vi "VI Linearisierung v2.vi"() -> ()   [LabVIEW 2020, in "Linearisierung v2.lvlib"] (continued)
              tunnel: w1175 -> [_ w1180]
              tunnel: w1170 -> [w1177 w1179]
              tunnel: [w1177 w1178] -> w1168
              frame False {
              }
              frame True {
                # "Zeilen von der Tabelle -1"
                n736 = call "Polynom Daten speichern.vi"("Aktionen"=Aktionen_Polynom_Daten_speichern."lesen") -> ("Aktiv"=w1187:bool[])  [unwired: 5 in, 5 out]
                n737 = Array Size(array=w1187) -> (size(s)=w1190:i32)
                n738 = Unbundle(w1179) -> ("Row"=w1193:u32, "Column"=w1192:u32)
                n739 = Subtract(x=w1190, y=29) -> (x-y=w1191:i32)
                n740 = Less Or Equal?(x=w1193, y=w1191) -> (x <= y?=w1194:bool)
                n741 = case shown="True" w1194 {
                  tunnel: w1193 -> [_ w1199]
                  tunnel: [w1197 w1199] -> w1181
                  tunnel: w1191 -> [w1197 _]
                  tunnel: w1192 -> [w1196 w1200]
                  tunnel: [w1195 w1198] -> w1178
                  frame False {
                    n742 = Bundle(w1197, "Column"=w1196) -> (w1195:cluster{i32, "Column":u32})  [unwired: 1 in]
                  }
                  frame True {
                    n743 = Bundle("Row"=w1199, "Column"=w1200) -> (w1198:cluster{"Row":u32, "Column":u32})  [unwired: 1 in]
                  }
                }
                n744 = property on="PolynomTabelleAnzeige" class="Tbl (strikt)"(error in=w1180, "Index Values"=w1178) -> (error out=w1183:errorcluster)  [unwired: 1 in, 1 out]
                n745 = property on="PolynomTabelleEingabe" class="Tbl (strikt)"(error in=w1180, "Index Values"=w1178) -> (error out=w1184:errorcluster)  [unwired: 1 in, 1 out]
                n746 = Build Array(w1181) -> (w1182:u32[])
                n747 = property on="PolynomAktiv" class="Arr"(error in=w1180, "Index Values"=w1182) -> (error out=w1185:errorcluster)  [unwired: 1 in, 1 out]
                n748 = Merge Errors(w1184, w1185, w1183) -> (w1186:errorcluster)
                n749 = call <vilib>:"Clear Errors.vi"("error in (no error)"=w1186) -> ()  [unwired: 5 in, 2 out]
              }
            }
          }
          frame "Spanfaktor" {
            # "#BugFix71"
            n750 = call "Spantabellenanzeige.vi"() -> ("SpanTabelle"=w1204:T48[][])  [unwired: 10 in, 1 out]
            n751 = property on="SpanTabelleEingabe" class="Tbl (strikt)"() -> (error out=w1207:errorcluster, "Index Values"=w1208:T176)  [unwired: 2 in, 1 out]
            n752 = Delete From Array(array=w1204, length=3 ("Länge"), index (col)=0 ("Deaktivierter Index (Spalte)")) -> (deleted portion=w1203:T48[][], array with subset deleted=w1202:T48[][])  [unwired: 1 in]
            n753 = local write "SpanTabelleAnzeige"(w1203) -> ()
            n754 = Not Equal?(x=w1212, y=w1208) -> (x != y?=w1211:cluster{"Row":bool, "Column":bool})
            n755 = Cluster To Array(cluster=w1211) -> (array=w1210:bool[])
            n756 = Or Array Elements(Boolean array=w1210) -> (logical OR=w1209:bool)
            n757 = case shown="True" w1209 {
              tunnel: w1208 -> [w1215 w1220]
              tunnel: w1207 -> [_ w1227]
              tunnel: w1202 -> [_ w1225]
              tunnel: [w1215 w1216] -> w1201
              frame False {
              }
              frame True {
                n758 = Array Size(array=w1225) -> (size(s)=w1219:i32[])
                n759 = Index Array(array=w1219) -> (element=w1218:i32)  [unwired: 1 in]
                n760 = local write "SpanTabelleEingabe"(w1225) -> ()
                n761 = Unbundle(w1220) -> ("Row"=w1223:u32, "Column"=w1222:u32)
                n762 = Subtract(x=w1218, y=29) -> (x-y=w1221:i32)
                n763 = Less Or Equal?(x=w1223, y=w1221) -> (x <= y?=w1224:bool)
                n764 = case shown="True" w1224 {
                  tunnel: w1223 -> [_ w1232]
                  tunnel: [w1230 w1232] -> _
                  tunnel: w1221 -> [w1230 _]
                  tunnel: w1222 -> [w1229 w1233]
                  tunnel: [w1228 w1231] -> w1216
                  frame False {
                    n765 = Bundle(w1230, "Column"=w1229) -> (w1228:cluster{i32, "Column":u32})  [unwired: 1 in]
                  }
                  frame True {
                    n766 = Bundle("Row"=w1232, "Column"=w1233) -> (w1231:cluster{"Row":u32, "Column":u32})  [unwired: 1 in]
                  }
                }
                n767 = property on="SpanTabelleEingabe" class="Tbl (strikt)"("Index Values"=w1216) -> ()  [unwired: 2 in, 2 out]
                n768 = property on="SpanTabelleAnzeige" class="Tbl (strikt)"(error in=w1227, "Index Values"=w1216) -> (error out=w1226:errorcluster)  [unwired: 1 in, 1 out]
                n769 = call <vilib>:"Clear Errors.vi"("error in (no error)"=w1226) -> ()  [unwired: 5 in, 2 out]
              }
            }
          }
        }
        n770 = call "FGV Gasteiler.vi"("Aktionen"=Aktionen_FGV_Gasteiler_Daten."lesen") -> ("Gasteiler Type"=w778:T15, "Anforderung"=w772:bool)  [unwired: 11 in, 6 out]
        n771 = local read "Gasteiler Type"() -> (w764:T15)
        n772 = call "FGV SpanEinstellungen.vi"("Aktion"=Aktion_FGV_SpanEinstellungen."lesen") -> ("automatisch out"=w783:T20)  [unwired: 6 in, 4 out]
        n773 = call "FGV Spans abarbeiten.vi"("Aktion"=Aktion_FGV_Spans_abarbeiten."lesen") -> ("running out"=w766:bool)  [unwired: 5 in, 5 out]
        n774 = call "LIN weiter schalten und Fehlerbehandlung.vi"("Anforderung in"=w772, "automatisch in"=w783, "TestRun"=w782, "Error in"=w770, "Gasteiler Type"=w778, "Referenzen Cluster"=w771, "get Test Data"=w769, "running in"=w766, "Beendet"=w781) -> ("Anforderung out"=w780:bool, "Gasteiler Type out"=w763:T15)  [unwired: 4 in, 1 out]
        n775 = Not Equal?(x=w763, y=w764) -> (x != y?=w765:bool)
        n776 = call "Test Status.vi"("LinV2 läuft"=w766, "Aktion"=Aktion_Test_Status."LinV2") -> ()  [unwired: 10 in, 4 out]
        n777 = case shown="True" w765 {
          tunnel: w763 -> [_ w815]
          frame False {
          }
          frame True {
            # "#HovaCAL_Interference_BugFixes"
            n778 = property on="Gasteiler Type" class="Ring (strikt)"("Val(Sgnl)"=w815) -> (error out=w816:errorcluster)  [unwired: 2 in, 1 out]
            n779 = call <vilib>:"Clear Errors.vi"("error in (no error)"=w816) -> ()  [unwired: 5 in, 2 out]
          }
        }
        n780 = case shown="True" w780 {
          tunnel: w763 -> [_ w823]
          frame False {
            n781 = local write "Störung Kommunikation"(FALSE) -> ()
            n782 = local write "Gasteilerstatus"("" ("Gasteilerstatus")) -> ()
          }
          frame True {
            # "GD Anforderung"
            n783 = case shown="4" w823 {
              frame 0, Default {
                # "LCD Touch Display"
                n784 = call "AK Komm.vi"("Aktionen"=Aktionen_AK_Komm."lesen") -> ("Error"=w826:T17, "Status"=→"Gasteilerstatus":string, "Störung Kommunikation"=w825:bool)  [unwired: 4 in, 4 out]
                "Störung Kommunikation" <- w825
                n785 = Unbundle By Name(w826) -> ("Pressure carrier gas"=w830:bool, "Pressure diluted gas"=w829:bool, "Outlet Pressure"=w828:bool, "SNOX before SAIR"=w827:bool)
                n786 = local write "Error"(w826) -> ()
                n787 = call "FGV Stoerungen sammeln und auswerten.vi"("Aktion"=Aktion_FGV_Stoerungen_sammeln_und_auswerten."lesen") -> ("Errors"=w831:T156)  [unwired: 12 in, 6 out]
                n788 = Bundle By Name(cluster=w831, "Störung Kommunikation"=w825, "Pressure carrier gas"=w830, "Pressure diluted gas"=w829, "Outlet Pressure"=w828, "SNOX before SAIR"=w827) -> (w824:T156)
                n789 = call "FGV Stoerungen sammeln und auswerten.vi"("Errors"=w824, "Aktion"=Aktion_FGV_Stoerungen_sammeln_und_auswerten."error") -> ()  [unwired: 11 in, 7 out]
              }
              frame 1 {
                # "Analog-Display"
                n790 = call "AK Komm_ALT.vi"("Aktionen_ALT"=Aktionen_AK_Komm_ALT."lesen") -> ("Error"=w841:T17, "Status"=w846:string, "Störung Kommunikation"=w842:bool)  [unwired: 6 in, 2 out]
                n791 = Unbundle By Name(w841) -> ("Pressure carrier gas"=w840:bool, "Pressure diluted gas"=w839:bool, "Outlet Pressure"=w838:bool, "SNOX before SAIR"=w837:bool)
                n792 = local write "Gasteilerstatus"(w846) -> ()
                n793 = local write "Störung Kommunikation"(w842) -> ()
                n794 = local write "Error"(w841) -> ()
                n795 = call "FGV Stoerungen sammeln und auswerten.vi"("Aktion"=Aktion_FGV_Stoerungen_sammeln_und_auswerten."lesen") -> ("Errors"=w843:T156)  [unwired: 12 in, 6 out]
                n796 = Bundle By Name(cluster=w843, "Störung Kommunikation"=w842, "Pressure carrier gas"=w840, "Pressure diluted gas"=w839, "Outlet Pressure"=w838, "SNOX before SAIR"=w837) -> (w836:T156)
                n797 = call "FGV Stoerungen sammeln und auswerten.vi"("Errors"=w836, "Aktion"=Aktion_FGV_Stoerungen_sammeln_und_auswerten."error") -> ()  [unwired: 11 in, 7 out]
              }
              frame 2 {
                # "AVL GDU"
                n798 = call "AK Komm.vi"("Aktionen"=Aktionen_AK_Komm."lesen") -> ("Error"=w850:T17, "Status"=w858:string, "Störung Kommunikation"=w849:bool)  [unwired: 4 in, 4 out]
                "Error" <- w850
                n799 = Unbundle By Name(w850) -> ("Pressure carrier gas"=w854:bool, "Pressure diluted gas"=w853:bool, "Outlet Pressure"=w852:bool, "SNOX before SAIR"=w851:bool)
                n800 = local write "Störung Kommunikation"(w849) -> ()
                n801 = local write "Gasteilerstatus"(w858) -> ()
                n802 = call "FGV Stoerungen sammeln und auswerten.vi"("Aktion"=Aktion_FGV_Stoerungen_sammeln_und_auswerten."lesen") -> ("Errors"=w855:T156)  [unwired: 12 in, 6 out]
                n803 = Bundle By Name(cluster=w855, "Störung Kommunikation"=w849, "Pressure carrier gas"=w854, "Pressure diluted gas"=w853, "Outlet Pressure"=w852, "SNOX before SAIR"=w851) -> (w848:T156)
                n804 = call "FGV Stoerungen sammeln und auswerten.vi"("Errors"=w848, "Aktion"=Aktion_FGV_Stoerungen_sammeln_und_auswerten."error") -> ()  [unwired: 11 in, 7 out]
              }
              frame 3 {
                # "Horiba GDC"
                n805 = call "GDC Kom.vi"("Befehl"=Aktion_Befehl."Alarm") -> ("Status (alarm)"=w861:bool, "Fehler"=w863:bool, "Status"=w864:string)  [unwired: 4 in, 4 out]
                "Störung Gasteiler" <- w861
                n806 = local write "Gasteilerstatus"(w864) -> ()
                n807 = local write "Störung Kommunikation"(w863) -> ()
                n808 = call "FGV Stoerungen sammeln und auswerten.vi"("Aktion"=Aktion_FGV_Stoerungen_sammeln_und_auswerten."lesen") -> ("Errors"=w862:T156)  [unwired: 12 in, 6 out]
                n809 = Bundle By Name(cluster=w862, "Störung Kommunikation"=w863, "Störung Gasteiler"=w861) -> (w860:T156)
                n810 = call "FGV Stoerungen sammeln und auswerten.vi"("Errors"=w860, "Aktion"=Aktion_FGV_Stoerungen_sammeln_und_auswerten."error") -> ()  [unwired: 11 in, 7 out]
              }
              frame 4 {
                # "#HovaCALErrors"
                n811 = call "FGV_HovaCAL_Interface_Kommandos.vi"("Aktion"=Aktion_FGV_HovaCAL_Interface_Kommandos."lesen") -> ("connected out ?"=w871:bool)  [unwired: 4 in, 5 out]
                n812 = Not(x=w871) -> (.not. x?=w872:bool)
                n813 = call "FGV Stoerungen sammeln und auswerten.vi"("Aktion"=Aktion_FGV_Stoerungen_sammeln_und_auswerten."lesen") -> ("Errors for AutoSPAN"=w868:T156)  [unwired: 12 in, 6 out]
                n814 = Unbundle By Name(w868) -> ("Störung Kommunikation"=w878:bool, "Pressure carrier gas"=w877:bool, "Pressure diluted gas"=w876:bool, "Outlet Pressure"=w875:bool)
                n815 = case shown="True" w872 {
                  selector: w872 -> [_ w881]
                  tunnel: w868 -> [_ w880]
                  frame False {
                  }
                  frame True {
                    n816 = Bundle By Name(cluster=w880, "Störung Kommunikation"=w881) -> (w882:T156)
                    n817 = call "FGV Stoerungen sammeln und auswerten.vi"("Errors"=w882, "Aktion"=Aktion_FGV_Stoerungen_sammeln_und_auswerten."error") -> ()  [unwired: 11 in, 7 out]
                  }
                }
                n818 = Or(x=w872, y=w878) -> (x .or. y?=w869:bool)
                "Störung Kommunikation 2" <- w869
                n819 = Bundle("Pressure carrier gas"=w877, "Pressure diluted gas"=w876, "Outlet Pressure"=w875, FALSE) -> (w870:T177)  [unwired: 1 in]
                "Error 2" <- w870
                n820 = local write "Störung Kommunikation"(w869) -> ()
                n821 = local write "Error"(w870) -> ()
              }
              frame 5 {
                # "manuell"
              }
            }
          }
        }
        n822 = call "Wertaenderung Systemeinstellungen.vi"("Aktion"=Aktion_Wertaenderung_Gasliste."lesen") -> ("Tests"=w794:T178)  [unwired: 13 in, 1 out]
        n823 = Unbundle By Name(w794) -> ("LinV2 läuft"=w793:bool)
        n824 = case shown="True" w793 {
          selector: w793 -> [_ w820]
          frame False {
          }
          frame True {
            n825 = property on="Systemeinstellung" class="Bool. (strikt)"("Val(Sgnl)"=w820) -> (error out=w819:errorcluster)  [unwired: 2 in, 1 out]
            n826 = call <vilib>:"Clear Errors.vi"("error in (no error)"=w819) -> ()  [unwired: 5 in, 2 out]
          }
        }
        n827 = call "Wertaenderung Gasliste.vi"("Aktion"=Aktion_Wertaenderung_Gasliste."lesen") -> ("Tests"=w791:T178)  [unwired: 13 in, 1 out]
        n828 = Unbundle By Name(w791) -> ("LinV2 läuft"=w790:bool)
        n829 = case shown="True" w790 {
          selector: w790 -> [_ w818]
          frame False {
          }
          frame True {
            n830 = property on="Gasliste geändert" class="Bool. (strikt)"("Val(Sgnl)"=w818) -> (error out=w817:errorcluster)  [unwired: 2 in, 1 out]
            n831 = call <vilib>:"Clear Errors.vi"("error in (no error)"=w817) -> ()  [unwired: 5 in, 2 out]
          }
        }
      }
      event Value Change {
        n832 = event-data() -> ()  [unwired: 1 in, 6 out]
        n833 = call "GD_MG_MagicFormula_OnOff.vi"("Aktion"=enum16{"lesen", "schreiben", "init"}."schreiben", "use old LNI"="use old LNI", "MG_use_magic_formula"="MG_use_magic_formula") -> ()  [unwired: 6 in, 2 out]
      }
      event "Systemeinstellung": Value Change {
        n834 = event-data() -> ()  [unwired: 1 in, 6 out]
        n835 = stacked-sequence {
          tunnel: w1242 -> [_ w1252 _]
          tunnel: w1241 -> [_ w1248 _]
          tunnel: w1240 -> [_ w1246 _]
          frame #0 {
            # "Bit wird von Systemeinstellungen gesetzt"
          }
          frame #1 {
            n836 = call "FGV Gasbottledefinition.vi"("Aktion"=Aktion_FGV_Gasbottledefinition."lesen") -> ("Gasflaschen Liste gesamt"=w1254:T105[])  [unwired: 8 in, 2 out]
            n837 = for {
              tunnel: w1254 -> [w1269]
              tunnel: w1252 -> [w1267] mode=indexing
              tunnel: [w1267] -> w1251 mode=indexing
              n838 = call "Gasflaschen Auswahl.vi"("Gasflaschen Liste gesamt"=w1269, "Ring (Eingang)"=w1267) -> ("error out"=w1268:errorcluster)  [unwired: 7 in, 2 out]
              n839 = call <vilib>:"Clear Errors.vi"("error in (no error)"=w1268) -> ()  [unwired: 5 in, 2 out]
            }
            n840 = call "Gasteiler initialisieren.vi"("Gasteiler Referenz"=w1246) -> ()  [unwired: 11 in]
            n841 = call "FGV SpanEinstellungen.vi"("Aktion"=Aktion_FGV_SpanEinstellungen."lesen") -> ("error out"=w1249:errorcluster, "SpanInletClusterArray out"=w1247:T19[])  [unwired: 6 in, 3 out]
            n842 = for {
              tunnel: w1248 -> [w1260] mode=indexing
              tunnel: w1247 -> [w1259] mode=indexing
              n843 = call "Analysator initialisieren.vi"("Referenz Analysator"=w1260) -> ("error out"=w1257:errorcluster, "Referenz Analysator out"=w1258:refnum<vi>)  [unwired: 9 in]
              n844 = Unbundle By Name(w1259) -> ("Analysator"=w1256:T21)
              n845 = property class="KombiFeld (strikt)"(reference=w1258, error in=w1257, "Value"=w1256) -> (error out=w1255:errorcluster)  [unwired: 1 out]
              n846 = call <vilib>:"Clear Errors.vi"("error in (no error)"=w1255) -> ()  [unwired: 5 in, 2 out]
            }
            n847 = for {
              tunnel: w1251 -> [w1265] mode=indexing
              tunnel: w1247 -> [w1264] mode=indexing
              shift-right: [w1262] -> _
              shift-left: w1249 -> [w1261]
              n848 = Unbundle By Name(w1264) -> ("Konfig Gasflasche"=w1263:T20)
              n849 = call "Konfig Gasflasche aktiv.vi"("error in (no error)"=w1261, "Konfig Gasflasche"=w1263, "Referenz Gasflasche"=w1265) -> ("error out"=w1266:errorcluster)  [unwired: 8 in]
              n850 = call <vilib>:"Clear Errors.vi"("error in (no error)"=w1266) -> ("error out"=w1262:errorcluster)  [unwired: 5 in, 1 out]
            }
          }
          frame #2 {
            n851 = call "Wertaenderung Systemeinstellungen.vi"("Aktion"=Aktion_Wertaenderung_Gasliste."LinV2 inaktiv") -> ()  [unwired: 13 in, 2 out]
            n852 = local write "Systemeinstellung"(FALSE ("Systemeinstellung")) -> ()
          }
        }
      }
      event "Gasliste geändert": Value Change {
        n853 = event-data() -> ()  [unwired: 1 in, 6 out]
        n854 = stacked-sequence {
          tunnel: w1276 -> [_ _ w1302 _]
          tunnel: w1275 -> [_ _ w1301 _]
          tunnel: w1274 -> [_ _ w1298 _]
          tunnel: w1273 -> [_ _ w1297 _]
          tunnel: [_ _ w1290 _] -> w1272
          frame #0 {
            # "Bit wird von Gasliste Vergleichen gesetzt"
          }
          frame #1 {
            n855 = call "FGV Gasliste.vi"("Aktionen"=FGV_FT-IR_Gasliste_Aktionen."lesen") -> ("Aktuelle Gasliste gesamt"=w1286:T48[])  [unwired: 8 in, 2 out]
            n856 = Build Array (concatenate)("---" ("String"), w1286) -> (w1279:T48[])
            n857 = call "Polynom Daten speichern.vi"("Aktionen"=Aktionen_Polynom_Daten_speichern."lesen") -> ("Aktiv"=w1282:bool[], "Namen"=w1284:string[])  [unwired: 5 in, 4 out]
            n858 = Build Array(w1279, w1284) -> (w1285:T48[][])
            n859 = call "FGV Komponentenreferenzen verwalten.vi"("Strings []"=w1279, "Aktion"=Aktion_FGV_Komponentenreferenz_verwalten."Ring beschreiben") -> ()  [unwired: 13 in, 1 out]
            n860 = Transpose 2D Array(2D array=w1285) -> (transposed array=w1283:T48[][])
            n861 = local write "PolynomAktiv"(w1282) -> ()
            n862 = local write "PolynomTabelleAnzeige"(w1283) -> ()
          }
          frame #2 {
            n863 = call "FGV Gasliste.vi"("Aktionen"=FGV_FT-IR_Gasliste_Aktionen."lesen") -> ("Aktuelle Gasliste gesamt"=w1289:T48[], "Aktuelle Gasliste FT-IR"=w1309:T48[])  [unwired: 8 in, 1 out]
            n864 = call "FT-IR EVID-Codes External Data.vi"("Aktionen"=Aktionen_EVID-Codes."lesen") -> ("Anzahl"=w1311:i32)  [unwired: 9 in, 5 out]
            n865 = Add(x=w1311, y=3) -> (x+y=w1303:i32)
            n866 = Array Size(array=w1309) -> (size(s)=w1308:i32)
            n867 = Array Size(array=w1289) -> (size(s)=w1304:i32)
            n868 = Subtract(x=w1308, y=w1303) -> (x-y=w1307:i32)
            n869 = Subtract(x=w1304, y=w1303) -> (x-y=w1300:i32)
            n870 = call "Zeile faerben.vi"("Anzahl"=w1307, "Table (Eingang)"=w1302) -> ("error out"=w1306:errorcluster)  [unwired: 9 in]
            n871 = call "Zeile faerben.vi"("error in (no error)"=w1306, "Anzahl"=w1307, "Table (Eingang)"=w1301) -> ("error out"=w1299:errorcluster)  [unwired: 8 in]
            n872 = call "Zeile faerben.vi"("error in (no error)"=w1299, "Anzahl"=w1300, "Table (Eingang)"=w1298) -> ("error out"=w1305:errorcluster)  [unwired: 8 in]
            n873 = call "Zeile faerben.vi"("error in (no error)"=w1305, "Anzahl"=w1300, "Table (Eingang)"=w1297) -> ()  [unwired: 8 in, 1 out]
            n874 = call "Tabelle in die einzelnen Seiten zerlegen.vi"("Aktion"=FGV_Aktion_Tabelle_zerlegen."vereinzeln", "Index (Seite)"=35) -> ("Sprachliste"=w1293:string[][])  [unwired: 7 in, 2 out]
            n875 = call "Texte in VIs uebersetzen.vi"("Sprachliste"=w1293, "String-Array zum Übersetzen"=w1289, "String zum Übersetzen"="Temp. Messzelle" ("Neues Element/Teil-Array")) -> ("String-Array zum Übersetzen"=w1292:string[], "String zum Übersetzen"=w1295:string)  [unwired: 8 in, 3 out]
            n876 = call "String in Array suchen.vi"("Nach String/Zeichen suchen (-)"=w1295, "String-Array"=w1292) -> ("Index"=w1290:i32)  [unwired: 7 in, 2 out]
          }
          frame #3 {
            n877 = call "Wertaenderung Gasliste.vi"("Aktion"=Aktion_Wertaenderung_Gasliste."LinV2 inaktiv") -> ()  [unwired: 13 in, 2 out]
            n878 = local write "Gasliste geändert"(FALSE ("Gasliste geändert")) -> ()
          }
        }
      }
      event Value Change {
        # "#HovaCALInterface"
        n879 = event-data() -> ()  [unwired: 1 in, 6 out]
        n880 = Build Array("MFC0", "MFC1", "MFC2", "MFC3", "MFC4") -> (w1317:T44[])
        n881 = flat-sequence {
          tunnel: w1317 -> [w1326]
          tunnel: w1323 -> [w1328]
          frame #0 {
            n882 = call "FGV_HovaCAL_Interface_SetData.vi"("Set Values Cluster in"=w1326, "Aktion"=Aktion_FGV_HovaCAL_Interface_SetData."Konzentrationen") -> ()  [unwired: 7 in, 7 out]
          }
          frame #1 {
            n883 = Select(t=Aktion_FGV_HovaCAL_Interface_Kommandos."on top" ("Aktion"), s=w1328, f=Aktion_FGV_HovaCAL_Interface_Kommandos."sammeln") -> (s? t:f=w1329:T79)
            n884 = call "FGV_HovaCAL_Interface_Kommandos.vi"("Aktion"=w1329, "Kommando in"=Aktion_FGV_HovaCAL_Interface_Kommunikation."Set Konzentrationen") -> ()  [unwired: 3 in, 6 out]
          }
        }
      }
      event Value Change {
        # "#HovaCALInterface"
        n885 = event-data() -> ("CtlRef"=w1336:refnum<vi>)  [unwired: 1 in]
        n886 = property class="Cluster"(reference=w1336) -> (error out=w1334:errorcluster, "Label.Text"=w1335:string)  [unwired: 1 in, 1 out]
        n887 = call <vilib>:"Clear Errors.vi"("error in (no error)"=w1334) -> ()  [unwired: 5 in, 2 out]
        n888 = case shown="\"HovaCAL Flow Input Cluster\"" w1335 {
          tunnel: w1337 -> [_ _ _ w1354 w1357]
          frame "False", Default {
          }
          frame "HovaCAL Flow AutoLin" {
            n889 = call "Lin Daten aufarbeiten.vi"("Aktionen"=Aktion_Lin_Daten_aufarbeiten."lesen") -> ("Lin-Polynom"=w1345:T119)  [unwired: 16 in, 10 out]
            n890 = Bundle By Name(cluster=w1345, "HovaCAL Flow AutoLin"="HovaCAL Flow AutoLin") -> (w1342:T119)
            n891 = call "Lin Daten aufarbeiten.vi"("Lin-Polynom"=w1342, "Aktionen"=Aktion_Lin_Daten_aufarbeiten."Protkolldaten") -> ("error out"=w1340:errorcluster)  [unwired: 15 in, 10 out]
            n892 = call "Lin Daten aufarbeiten.vi"("error in (no error)"=w1340, "Aktionen"=Aktion_Lin_Daten_aufarbeiten."speichern") -> ()  [unwired: 15 in, 11 out]
          }
          frame "Pump state for LIN" {
            n893 = call "Lin Daten aufarbeiten.vi"("Aktionen"=Aktion_Lin_Daten_aufarbeiten."lesen") -> ("Lin-Polynom"=w1352:T119)  [unwired: 16 in, 10 out]
            n894 = Bundle By Name(cluster=w1352, "MFC Output"="Pump state for LIN") -> (w1350:T119)
            n895 = call "Lin Daten aufarbeiten.vi"("Lin-Polynom"=w1350, "Aktionen"=Aktion_Lin_Daten_aufarbeiten."Protkolldaten") -> ("error out"=w1348:errorcluster)  [unwired: 15 in, 10 out]
            n896 = call "Lin Daten aufarbeiten.vi"("error in (no error)"=w1348, "Aktionen"=Aktion_Lin_Daten_aufarbeiten."speichern") -> ()  [unwired: 15 in, 11 out]
          }
          frame "HovaCAL SetPumpMode" {
            n897 = Unbundle By Name("HovaCAL SetPumpMode") -> ("Run"=w1355:bool)
            n898 = call "HovaCAL_Interface_SetPumpRun.vi"("sofort"=w1354, "run"=w1355) -> ()  [unwired: 9 in, 1 out]
          }
          frame "HovaCAL Flow Input Cluster" {
            n899 = Unbundle By Name("HovaCAL Flow Input Cluster") -> ("HovaCAL Flow Input Cluster"=w1358:dbl)
            n900 = call "HovaCAL_Interface_SetFlow.vi"("sofort"=w1357, "total flow setpoint"=w1358) -> ()  [unwired: 9 in, 1 out]
          }
        }
      }
      event Value Change {
        # "#HovaCALInterface"
        n901 = event-data() -> ()  [unwired: 1 in, 6 out]
        n902 = flat-sequence {
          tunnel: "HovaCAL Temperature" -> [w1365]
          tunnel: w1361 -> [w1367]
          frame #0 {
            n903 = call "FGV_HovaCAL_Interface_SetData.vi"("Temperature"=w1365, "Aktion"=Aktion_FGV_HovaCAL_Interface_SetData."Temperaturen") -> ()  [unwired: 7 in, 7 out]
          }
          frame #1 {
            n904 = Select(t=Aktion_FGV_HovaCAL_Interface_Kommandos."on top" ("Aktion"), s=w1367, f=Aktion_FGV_HovaCAL_Interface_Kommandos."sammeln") -> (s? t:f=w1368:T79)
            n905 = call "FGV_HovaCAL_Interface_Kommandos.vi"("Aktion"=w1368, "Kommando in"=Aktion_FGV_HovaCAL_Interface_Kommunikation."Set Temperaturen") -> ()  [unwired: 3 in, 6 out]
          }
        }
      }
      event Value Change {
        # "#HovaCALInterface"
        n906 = event-data() -> ()  [unwired: 1 in, 1 out]
        n907 = call "Pump Concentrations in ppm.vi"("Pump Concetration in"="Pump 1") -> ("Pump Concentration out"=w1376:T167)  [unwired: 10 in]
        n908 = call "Pump Concentrations in ppm.vi"("Pump Concetration in"="Pump 2") -> ("Pump Concentration out"=w1373:T167)  [unwired: 10 in]
        n909 = Build Array(w1376, w1373) -> (w1377:T167[])
        n910 = flat-sequence {
          tunnel: w1377 -> [w1381]
          tunnel: w1378 -> [w1383]
          frame #0 {
            n911 = call "FGV_HovaCAL_Interface_SetData.vi"("Pump Concentrations-Cluster"=w1381, "Aktion"=Aktion_FGV_HovaCAL_Interface_SetData."Pumpe Konzentration") -> ()  [unwired: 7 in, 7 out]
          }
          frame #1 {
            n912 = Select(t=Aktion_FGV_HovaCAL_Interface_Kommandos."on top" ("Aktion"), s=w1383, f=Aktion_FGV_HovaCAL_Interface_Kommandos."sammeln") -> (s? t:f=w1384:T79)
            n913 = call "FGV_HovaCAL_Interface_Kommandos.vi"("Aktion"=w1384, "Kommando in"=Aktion_FGV_HovaCAL_Interface_Kommunikation."Set Pumpe Konzenration") -> ()  [unwired: 3 in, 6 out]
          }
        }
      }
      event Value Change {
        # "#HovaCALInterface"
        n914 = event-data() -> ()  [unwired: 1 in, 6 out]
        n915 = flat-sequence {
          tunnel: "HovaCAL SetPumpMode-Cluster" -> [w1393]
          tunnel: w1389 -> [w1395]
          frame #0 {
            n916 = call "FGV_HovaCAL_Interface_SetData.vi"("PumpMode-Cluster in"=w1393, "Aktion"=Aktion_FGV_HovaCAL_Interface_SetData."Pumpen Parameter") -> ()  [unwired: 7 in, 7 out]
          }
          frame #1 {
            n917 = Select(t=Aktion_FGV_HovaCAL_Interface_Kommandos."on top" ("Aktion"), s=w1395, f=Aktion_FGV_HovaCAL_Interface_Kommandos."sammeln") -> (s? t:f=w1396:T79)
            n918 = call "FGV_HovaCAL_Interface_Kommandos.vi"("Aktion"=w1396, "Kommando in"=Aktion_FGV_HovaCAL_Interface_Kommunikation."Set Pumpen Parameter") -> ()  [unwired: 3 in, 6 out]
          }
        }
      }
      event Value Change {
        # "#HovaCALInterface"
        n919 = event-data() -> ()  [unwired: 1 in, 6 out]
        n920 = flat-sequence {
          tunnel: "HovaCAL Cluster.PumpModeGeneral" -> [w1405]
          tunnel: w1401 -> [w1407]
          frame #0 {
            n921 = call "FGV_HovaCAL_Interface_SetData.vi"("PumpModeGeneral-Cluster in"=w1405, "Aktion"=Aktion_FGV_HovaCAL_Interface_SetData."Pumpe run") -> ()  [unwired: 7 in, 7 out]
          }
          frame #1 {
            n922 = Select(t=Aktion_FGV_HovaCAL_Interface_Kommandos."on top" ("Aktion"), s=w1407, f=Aktion_FGV_HovaCAL_Interface_Kommandos."sammeln") -> (s? t:f=w1408:T79)
            n923 = call "FGV_HovaCAL_Interface_Kommandos.vi"("Aktion"=w1408, "Kommando in"=Aktion_FGV_HovaCAL_Interface_Kommunikation."Set Pumpe run") -> ()  [unwired: 3 in, 6 out]
          }
        }
      }
      event Value Change {
        # "#HovaCALInterface"
        n924 = event-data() -> ()  [unwired: 1 in, 6 out]
        n925 = Build Array("HovaCAL MFC Gase Cluster 1", "HovaCAL MFC Gase Cluster 2", "HovaCAL MFC Gase Cluster 3", "HovaCAL MFC Gase Cluster 4", "HovaCAL MFC Gase Cluster 5") -> (w1413:T46[])
        n926 = flat-sequence {
          tunnel: w1413 -> [w1423]
          tunnel: w1419 -> [w1425]
          frame #0 {
            n927 = call "Set MFC Gase.vi"("HovaCAL MFC Gase Cluster"=w1423) -> ("mfc Gasnamen out"=w1422:string[])  [unwired: 9 in, 1 out]
            n928 = call "FGV_HovaCAL_Interface_MFC_Gase.vi"("Aktion"=Aktion_FGV_HovaCAL_Interface_Gasliste."setzen", "mfc Gasnamen in"=w1422) -> ()  [unwired: 7 in, 3 out]
          }
          frame #1 {
            n929 = Select(t=Aktion_FGV_HovaCAL_Interface_Kommandos."on top" ("Aktion"), s=w1425, f=Aktion_FGV_HovaCAL_Interface_Kommandos."sammeln") -> (s? t:f=w1426:T79)
            n930 = call "FGV_HovaCAL_Interface_Kommandos.vi"("Aktion"=w1426, "Kommando in"=Aktion_FGV_HovaCAL_Interface_Kommunikation."Set Gase") -> ()  [unwired: 3 in, 6 out]
          }
        }
      }
      event Value Change {
        # "#HovaCALInterface"
        n931 = event-data() -> ()  [unwired: 1 in, 6 out]
        n932 = flat-sequence {
          tunnel: "HovaCAL Limits Cluster" -> [w1435]
          tunnel: w1431 -> [w1437]
          frame #0 {
            n933 = call "FGV_HovaCAL_Interface_SetData.vi"("Aktion"=Aktion_FGV_HovaCAL_Interface_SetData."Limits", "Limits Cluster in"=w1435) -> ()  [unwired: 7 in, 7 out]
          }
          frame #1 {
            n934 = Select(t=Aktion_FGV_HovaCAL_Interface_Kommandos."on top" ("Aktion"), s=w1437, f=Aktion_FGV_HovaCAL_Interface_Kommandos."sammeln") -> (s? t:f=w1438:T79)
            n935 = call "FGV_HovaCAL_Interface_Kommandos.vi"("Aktion"=w1438, "Kommando in"=Aktion_FGV_HovaCAL_Interface_Kommunikation."Set Limits") -> ()  [unwired: 3 in, 6 out]
          }
        }
      }
      event Value Change {
        n936 = event-data() -> ()  [unwired: 1 in, 6 out]
        n937 = call "FGV_HovaCAL_Interface_Kommandos.vi"("Aktion"=Aktion_FGV_HovaCAL_Interface_Kommandos."freigeben") -> ()  [unwired: 4 in, 6 out]
      }
      event Value Change {
        n938 = event-data() -> ()  [unwired: 1 in, 6 out]
        n939 = call "FGV SystemEinstellungenV2.vi"("Aktion"=Aktion_FGV_SystemEinstellungenV2."lesen") -> ("Gasteiler"=w1455:T180)  [unwired: 5 in, 5 out]
        n940 = Unbundle By Name(w1455) -> ("GasteilerDefinitionsListe"=w1454:T179[])
        n941 = Index Array(array=w1454, index="Konfig Gasteiler") -> (element=w1449:T179)
        n942 = Bundle By Name(cluster=T118 {"Gasteiler"="", "Gasteiler Stufen"=128, "Gasteiler Type"=0, "Konfig Gasteiler"=10000, "Gasteiler Span Eingänge"=128} ("Gasteiler Daten"), "Konfig Gasteiler"="Konfig Gasteiler") -> (w1450:T118)
        n943 = Unbundle By Name(w1449) -> ("Gasteiler Type"=w1453:string)
        n944 = property on="Gasteiler" class="Str (strikt)"("Val(Sgnl)"=w1453) -> (error out=w1452:errorcluster)  [unwired: 2 in, 1 out]
        n945 = call "FGV Gasteiler.vi"("Gasteiler Daten"=w1450, "Aktionen"=Aktionen_FGV_Gasteiler_Daten."Gasteiler Daten") -> ()  [unwired: 10 in, 8 out]
        n946 = call <vilib>:"Clear Errors.vi"("error in (no error)"=w1452) -> ()  [unwired: 5 in, 2 out]
      }
      event "SpanTabelleEingabe": Value Change {
        n947 = event-data() -> ("OldVal"=w1465:string[][], "NewVal"=w1464:string[][])  [unwired: 1 in]
        n948 = for {
          tunnel: w1465 -> [w1472] mode=indexing
          tunnel: w1464 -> [w1471] mode=indexing
          tunnel: [w1469] -> w1461
          tunnel: [w1468] -> w1462
          i -> [w1469]
          stop <- w1470 stop-if-true
          n949 = for {
            tunnel: w1472 -> [w1476] mode=indexing
            tunnel: w1471 -> [w1475] mode=indexing
            tunnel: [w1474] -> w1470
            tunnel: [w1473] -> w1468
            i -> [w1473]
            stop <- w1474 stop-if-true
            n950 = Not Equal?(x=w1476, y=w1475) -> (x != y?=w1474:bool)
          }
        }
        n951 = Index Array(array="SpanTabelleEingabe", index (row)=w1461, index (col)=w1462) -> (element=w1460:string)
        n952 = case shown="0" w1462 {
          tunnel: w1461 -> [_ w1478 w1482]
          tunnel: w1460 -> [_ w1477 w1481]
          frame 7, Default {
          }
          frame 0 {
            n953 = Add(x=9000 ("Feedback"), y=w1478) -> (x+y=w1480:i32)
            n954 = call "TOOLweb SET.vi"("Wert-String"=w1477, "EVID-Nummer"=w1480) -> ()  [unwired: 3 in, 3 out]
          }
          frame 1 {
            n955 = Add(x=9500 ("Feedback"), y=w1482) -> (x+y=w1484:i32)
            n956 = call "TOOLweb SET.vi"("Wert-String"=w1481, "EVID-Nummer"=w1484) -> ()  [unwired: 3 in, 3 out]
          }
        }
      }
      event Value Change {
        n957 = event-data() -> ()  [unwired: 1 in, 1 out]
        n958 = case shown="True" "PMD kalibrieren" {
          tunnel: w1488 -> [_ w1505]
          frame False {
          }
          frame True {
            n959 = call "FGV-Funktionstasten.vi"("Herkunft"="Linearisierung PMA", "Zustand"=Zustaende."Kalibrieren", "Aktion"=Funktionstasten-Aktion."Zustand setzen") -> ()  [unwired: 5 in, 8 out]
            n960 = local read "Status kalibrieren"() -> (w1510:string)
            n961 = call "Texte in VIs uebersetzen.vi"("Sprachliste"=w1505, "String zum Übersetzen"="PMD Kalibrieren.\nAutoKal PMD gestartet." ("String")) -> ("String zum Übersetzen"=w1506:string)  [unwired: 9 in, 4 out]
            n962 = Concatenate Strings(w1510, "\r", w1506) -> (w1509:string)
            n963 = local write "Status kalibrieren"(w1509) -> ()
          }
        }
        n964 = case shown="True" "FTIR Kalibrieren" {
          tunnel: w1488 -> [_ w1492]
          frame False {
          }
          frame True {
            n965 = control-ref of="Anforderung"() -> (w1495:refnum<vi>)
            n966 = control-ref of="Status kalibrieren"() -> (w1494:refnum<vi>)
            n967 = call "FT-IR Kalibrieren Linearisierung.vi"("Kalibrier Optionen:"="Kalibrier Optionen:", "Sprachliste"=w1492, "reference (Eingang)"=w1495, "String (Eingang)"=w1494) -> ()  [unwired: 8 in]
          }
        }
        n968 = case shown="True" "FID kalibrieren" {
          tunnel: w1488 -> [_ w1496]
          frame False {
          }
          frame True {
            n969 = call "FGV-Funktionstasten.vi"("Herkunft"="Linearisierung FID", "Zustand"=Zustaende."Kalibrieren", "Aktion"=Funktionstasten-Aktion."Zustand setzen") -> ()  [unwired: 5 in, 8 out]
            n970 = local read "Status kalibrieren"() -> (w1501:string)
            n971 = call "Texte in VIs uebersetzen.vi"("Sprachliste"=w1496, "String zum Übersetzen"="FID Kalibrieren.\nAutoKal FID gestartet." ("String")) -> ("String zum Übersetzen"=w1497:string)  [unwired: 9 in, 4 out]
            n972 = Concatenate Strings(w1501, "\r", w1497) -> (w1500:string)
            n973 = local write "Status kalibrieren"(w1500) -> ()
          }
        }
      }
      event Value Change {
        # "Wenn Komponente THC dann FID\nWenn Komponente O2 dann PMA\nalles andere = FTIR"
        n974 = event-data() -> ()  [unwired: 1 in, 1 out]
        n975 = call "Lin Daten aufarbeiten.vi"("Aktionen"=Aktion_Lin_Daten_aufarbeiten."lesen") -> ("Lin-Polynom"=w1526:T119)  [unwired: 16 in, 10 out]
        n976 = control-ref of="Boolsch für LinStart"() -> (w1515:refnum<vi>)
        n977 = Unbundle By Name(w1526) -> ("Komponentenauswahl"=w1527:T120, "Gasnummer:"=w1528:u8)
        n978 = call "FGV Autokal GT.vi"("Aktion FGV AutoKal"=Aktion_FGV_Autokal_GT."Referenz Start", "Start LinCheck"=w1515) -> ()  [unwired: 7 in, 3 out]
        n979 = Index Array(array=w1527, index=w1528) -> (element=w1529:cluster{"Komponente:":T7, "Konzentration":dbl})
        n980 = Unbundle By Name(w1529) -> ("Komponente:"=w1519:T7)
        n981 = Decrement(x=w1519) -> (x-1=w1517:T7)
        n982 = call "FGV Gasliste.vi"("Aktionen"=FGV_FT-IR_Gasliste_Aktionen."lesen") -> ("Aktuelle Gasliste gesamt"=w1521:T48[])  [unwired: 8 in, 2 out]
        n983 = for {
          tunnel: w1521 -> [w1539]
          tunnel: string[] ["O2_", "THC_", "FT-IR"] ("String-Array") -> [w1538] mode=indexing
          tunnel: w1517 -> [w1536]
          tunnel: [w1535] -> w1518
          i -> [w1535]
          stop <- w1534 stop-if-true
          n984 = call "String in Array suchen.vi"("Nach String/Zeichen suchen (-)"=w1538, "String-Array"=w1539) -> ("Index"=w1537:i32)  [unwired: 7 in, 2 out]
          n985 = Equal?(x=w1537, y=w1536) -> (x = y?=w1534:bool)
        }
        n986 = case shown="2, Standard" w1518 {
          tunnel: [TRUE _ _] -> w1522
          tunnel: [_ TRUE _] -> w1524
          tunnel: [_ _ TRUE] -> w1523
          frame 0 {
          }
          frame 1 {
          }
          frame 2, Default {
          }
        }
        n987 = case shown="True" w1522 {
          tunnel: w1532 -> [_ w1556]
          frame False {
          }
          frame True {
            n988 = call "FGV-Funktionstasten.vi"("Herkunft"="Linearisierung PMA GT", "Zustand"=Zustaende."Kalibrieren", "Aktion"=Funktionstasten-Aktion."Zustand setzen") -> ()  [unwired: 5 in, 8 out]
            n989 = local read "Status kalibrieren"() -> (w1561:string)
            n990 = call "Texte in VIs uebersetzen.vi"("Sprachliste"=w1556, "String zum Übersetzen"="PMD Kalibrieren.\nAutoKal PMD gestartet." ("String")) -> ("String zum Übersetzen"=w1557:string)  [unwired: 9 in, 4 out]
            n991 = Concatenate Strings(w1561, "\r", w1557) -> (w1560:string)
            n992 = local write "Status kalibrieren"(w1560) -> ()
          }
        }
        n993 = case shown="True" w1524 {
          tunnel: w1532 -> [_ w1547]
          frame False {
          }
          frame True {
            n994 = call "FGV-Funktionstasten.vi"("Herkunft"="Linearisierung FID GT", "Zustand"=Zustaende."Kalibrieren", "Aktion"=Funktionstasten-Aktion."Zustand setzen") -> ()  [unwired: 5 in, 8 out]
            n995 = local read "Status kalibrieren"() -> (w1552:string)
            n996 = call "Texte in VIs uebersetzen.vi"("Sprachliste"=w1547, "String zum Übersetzen"="FID Kalibrieren.\nAutoKal FID gestartet." ("String")) -> ("String zum Übersetzen"=w1548:string)  [unwired: 9 in, 4 out]
            n997 = Concatenate Strings(w1552, "\r", w1548) -> (w1551:string)
            n998 = local write "Status kalibrieren"(w1551) -> ()
          }
        }
        n999 = case shown="True" w1523 {
          tunnel: w1532 -> [_ w1546]
          frame False {
          }
          frame True {
            n1000 = control-ref of="Anforderung"() -> (w1543:refnum<vi>)
            n1001 = control-ref of="Status kalibrieren"() -> (w1544:refnum<vi>)
            n1002 = local read "Kalibrier Optionen:"() -> (w1545:enum32{"Gasteiler", "ohne Gasteiler", "PNS"})
            n1003 = call "FT-IR Kalibrieren Linearisierung.vi"("Kalibrier Optionen:"=w1545, "Sprachliste"=w1546, "reference (Eingang)"=w1543, "String (Eingang)"=w1544) -> ()  [unwired: 8 in]
          }
        }
      }
      event Value Change {
        n1004 = event-data() -> ()  [unwired: 1 in, 1 out]
        n1005 = local read "Kalibrier Optionen:"() -> (w1568:enum32{"Gasteiler", "ohne Gasteiler", "PNS"})
        n1006 = case shown="True" "FID E kalibrieren" {
          tunnel: w1568 -> [_ w1609]
          tunnel: w1567 -> [_ w1608]
          frame False {
          }
          frame True {
            n1007 = case shown="\"Gasteiler\", Standard" w1609 {
              tunnel: w1608 -> [w1610 _ _]
              frame "Gasteiler", Default {
                n1008 = stacked-sequence {
                  tunnel: w1610 -> [w1611 _ _ _]
                  frame #0 {
                    n1009 = local read "Anforderung"() -> (w1612:T4)
                    n1010 = case shown="True" w1612 {
                      tunnel: w1611 -> [w1613 w1619]
                      frame False {
                        n1011 = local read "Status kalibrieren"() -> (w1616:string)
                        n1012 = call "Texte in VIs uebersetzen.vi"("Sprachliste"=w1613, "String zum Übersetzen"="Keine Anforderung Gasteiler!\nGas manuell aufschalten!" ("String")) -> ("String zum Übersetzen"=w1614:string)  [unwired: 9 in, 4 out]
                        n1013 = Concatenate Strings(w1616, "\r", w1614) -> (w1617:string)
                        n1014 = local write "Status kalibrieren"(w1617) -> ()
                      }
                      frame True {
                        n1015 = local read "Status kalibrieren"() -> (w1624:string)
                        n1016 = call "Gasteiler_Endpunkt.vi"() -> ()  [unwired: 12 in]
                        n1017 = call "Texte in VIs uebersetzen.vi"("Sprachliste"=w1619, "String zum Übersetzen"="E-Gas am Gasteiler aufgeschalten." ("String")) -> ("String zum Übersetzen"=w1620:string)  [unwired: 9 in, 4 out]
                        n1018 = Concatenate Strings(w1624, "\r", w1620) -> (w1623:string)
                        n1019 = local write "Status kalibrieren"(w1623) -> ()
                      }
                    }
                  }
                  frame #1 {
                    n1020 = call "FGV-Funktionstasten.vi"("Herkunft"="Linearisierung", "Zustand"=Zustaende."Cal-Gas", "Aktion"=Funktionstasten-Aktion."Zustand setzen") -> ()  [unwired: 5 in, 8 out]
                  }
                  frame #2 {
                    n1021 = call "FID Manuell Kalibrieren.vi"("über GT"=TRUE, "Kalibrieren"=FID_Kalibrieren."THC Endpunkt") -> ()  [unwired: 8 in, 2 out]
                  }
                  frame #3 {
                    n1022 = call "FGV-Funktionstasten.vi"("Herkunft"="Linearisierung", "Zustand"=Zustaende."Standby", "Aktion"=Funktionstasten-Aktion."Zustand setzen") -> ()  [unwired: 5 in, 8 out]
                    n1023 = call "Gasteiler_Standby.vi"() -> ()  [unwired: 12 in]
                  }
                }
              }
              frame "PNS" {
                n1024 = flat-sequence {
                  frame #0 {
                    n1025 = call "FGV-Funktionstasten.vi"("Herkunft"="Linearisierung", "Zustand"=Zustaende."Cal-Gas", "Aktion"=Funktionstasten-Aktion."Zustand setzen") -> ()  [unwired: 5 in, 8 out]
                  }
                  frame #1 {
                    n1026 = call "FID Manuell Kalibrieren.vi"("Kalibrieren"=FID_Kalibrieren."THC Endpunkt") -> ()  [unwired: 9 in, 2 out]
                  }
                  frame #2 {
                    n1027 = call "FGV-Funktionstasten.vi"("Herkunft"="Linearisierung", "Zustand"=Zustaende."Standby", "Aktion"=Funktionstasten-Aktion."Zustand setzen") -> ()  [unwired: 5 in, 8 out]
                  }
                }
              }
              frame "ohne Gasteiler" {
                n1028 = flat-sequence {
                  frame #0 {
                    n1029 = call "FGV-Funktionstasten.vi"("Herkunft"="Linearisierung", "Zustand"=Zustaende."0-Gas", "Aktion"=Funktionstasten-Aktion."Zustand setzen") -> ()  [unwired: 5 in, 8 out]
                  }
                  frame #1 {
                    n1030 = call "FID Manuell Kalibrieren.vi"("Kalibrieren"=FID_Kalibrieren."THC Endpunkt") -> ()  [unwired: 9 in, 2 out]
                  }
                  frame #2 {
                    n1031 = call "FGV-Funktionstasten.vi"("Herkunft"="Linearisierung", "Zustand"=Zustaende."Standby", "Aktion"=Funktionstasten-Aktion."Zustand setzen") -> ()  [unwired: 5 in, 8 out]
                  }
                }
              }
            }
          }
        }
        n1032 = case shown="True" "PMD 0 kalibrieren" {
          tunnel: w1567 -> [_ w1686]
          tunnel: w1568 -> [_ w1685]
          frame False {
          }
          frame True {
            n1033 = case shown="\"Gasteiler\", Standard" w1685 {
              tunnel: w1686 -> [w1687 _ _]
              frame "Gasteiler", Default {
                n1034 = stacked-sequence {
                  tunnel: w1687 -> [w1688 _ _ _]
                  frame #0 {
                    n1035 = local read "Anforderung"() -> (w1689:T4)
                    n1036 = case shown="False" w1689 {
                      tunnel: w1688 -> [w1690 _]
                      frame False {
                        n1037 = local read "Status kalibrieren"() -> (w1695:string)
                        n1038 = call "Texte in VIs uebersetzen.vi"("Sprachliste"=w1690, "String zum Übersetzen"="Keine Anforderung Gasteiler!\n0-Gas manuell aufschalten!" ("String")) -> ("String zum Übersetzen"=w1691:string)  [unwired: 9 in, 4 out]
                        n1039 = Concatenate Strings(w1695, "\r", w1691) -> (w1694:string)
                        n1040 = local write "Status kalibrieren"(w1694) -> ()
                      }
                      frame True {
                        n1041 = call "Gasteiler_Nullpunkt.vi"() -> ()  [unwired: 12 in]
                      }
                    }
                  }
                  frame #1 {
                    n1042 = call "FGV-Funktionstasten.vi"("Herkunft"="Linearisierung", "Zustand"=Zustaende."Cal-Gas", "Aktion"=Funktionstasten-Aktion."Zustand setzen") -> ()  [unwired: 5 in, 8 out]
                  }
                  frame #2 {
                    n1043 = call "PMA Manuell Kalibrieren.vi"("Kalibrieren"=Kalibrierung_O2."Nullpunkt O2") -> ()  [unwired: 9 in, 2 out]
                  }
                  frame #3 {
                    n1044 = call "Gasteiler_Standby.vi"() -> ()  [unwired: 12 in]
                    n1045 = call "FGV-Funktionstasten.vi"("Herkunft"="Linearisierung", "Zustand"=Zustaende."Standby", "Aktion"=Funktionstasten-Aktion."Zustand setzen") -> ()  [unwired: 5 in, 8 out]
                  }
                }
              }
              frame "PNS" {
                n1046 = flat-sequence {
                  frame #0 {
                    n1047 = call "FGV-Funktionstasten.vi"("Herkunft"="Linearisierung", "Zustand"=Zustaende."Cal-Gas", "Aktion"=Funktionstasten-Aktion."Zustand setzen") -> ()  [unwired: 5 in, 8 out]
                  }
                  frame #1 {
                    n1048 = call "PMA Manuell Kalibrieren.vi"("Kalibrieren"=Kalibrierung_O2."Nullpunkt O2") -> ()  [unwired: 9 in, 2 out]
                  }
                  frame #2 {
                    n1049 = call "FGV-Funktionstasten.vi"("Herkunft"="Linearisierung", "Zustand"=Zustaende."Standby", "Aktion"=Funktionstasten-Aktion."Zustand setzen") -> ()  [unwired: 5 in, 8 out]
                  }
                }
              }
              frame "ohne Gasteiler" {
                n1050 = flat-sequence {
                  frame #0 {
                    n1051 = call "FGV-Funktionstasten.vi"("Herkunft"="Linearisierung", "Zustand"=Zustaende."0-Gas", "Aktion"=Funktionstasten-Aktion."Zustand setzen") -> ()  [unwired: 5 in, 8 out]
                  }
                  frame #1 {
                    n1052 = call "PMA Manuell Kalibrieren.vi"("Kalibrieren"=Kalibrierung_O2."Nullpunkt O2") -> ()  [unwired: 9 in, 2 out]
                  }
                  frame #2 {
                    n1053 = call "FGV-Funktionstasten.vi"("Herkunft"="Linearisierung", "Zustand"=Zustaende."Standby", "Aktion"=Funktionstasten-Aktion."Zustand setzen") -> ()  [unwired: 5 in, 8 out]
                  }
                }
              }
            }
          }
        }
        n1054 = case shown="True" "FID 0 kalibrieren" {
          tunnel: w1568 -> [_ w1648]
          tunnel: w1567 -> [_ w1647]
          frame False {
          }
          frame True {
            n1055 = case shown="\"Gasteiler\", Standard" w1648 {
              tunnel: w1647 -> [w1649 _ _]
              frame "Gasteiler", Default {
                n1056 = stacked-sequence {
                  tunnel: w1649 -> [w1650 _ _ _]
                  frame #0 {
                    n1057 = local read "Anforderung"() -> (w1651:T4)
                    n1058 = case shown="True" w1651 {
                      tunnel: w1650 -> [w1652 w1658]
                      frame False {
                        n1059 = local read "Status kalibrieren"() -> (w1657:string)
                        n1060 = call "Texte in VIs uebersetzen.vi"("Sprachliste"=w1652, "String zum Übersetzen"="Keine Anforderung Gasteiler!\n0-Gas manuell aufschalten!" ("String")) -> ("String zum Übersetzen"=w1653:string)  [unwired: 9 in, 4 out]
                        n1061 = Concatenate Strings(w1657, "\r", w1653) -> (w1656:string)
                        n1062 = local write "Status kalibrieren"(w1656) -> ()
                      }
                      frame True {
                        n1063 = local read "Status kalibrieren"() -> (w1663:string)
                        n1064 = call "Gasteiler_Nullpunkt.vi"() -> ()  [unwired: 12 in]
                        n1065 = call "Texte in VIs uebersetzen.vi"("Sprachliste"=w1658, "String zum Übersetzen"="0-Gas am Gasteiler aufgeschalten" ("String")) -> ("String zum Übersetzen"=w1659:string)  [unwired: 9 in, 4 out]
